vi "FFT no clk.vi"() -> ()   [LabVIEW 2014]
uses:
  <vilib>/Platform/TimedLoop/XDataNode/timing_clust.ctl
  <vilib>/Platform/TimedLoop/XDataNode/nitl_modes.ctl
  <vilib>/Platform/TimedLoop/XDataNode/wakeup.ctl
  <vilib>/rvi/Analysis/measure/FFT/simModelSupport/niFPGA FFT Streaming Sim Properties.ctl
  <vilib>/rvi/Analysis/measure/FFT/simModelSupport/niFPGA FFT Sim Stream Group Properties.ctl
  <vilib>/rvi/Analysis/measure/FFT/simModelSupport/niFPGA FFT Sim Types.ctl
  <vilib>/rvi/Analysis/measure/FFT/simModelSupport/niFpgaFFTSimArithmeticProperties.ctl
  <vilib>/rvi/Analysis/measure/FFT/simModelSupport/niFpgaFFTSimDfxp.ctl
  <vilib>/fxp/LVFixedPointQuantizationPolicyTypeDef.ctl
  <vilib>/rvi/Analysis/measure/FFT/XNode/niFpgaFFTButterflyDelays.ctl
  <vilib>/rvi/Emulation/niFpgaSctlEmulationGetInTimedLoop.vi
  <vilib>/rvi/Emulation/niFpgaEmulationReportErrorSimple.vi
  <vilib>/rvi/Emulation/niFpgaGetClockAttributes.vi
  <vilib>/rvi/Emulation/niFpgaCriticalErrorInLSC.vi
  <vilib>/rvi/Emulation/niFpgaEmulationIsFPGAContextNoSignature.vi
  <vilib>/rvi/errors/niFpgaSetErrorForExecOnDevCompSimple.vi
  <vilib>/rvi/eio/common/nirviEmuReportErrorAndStop.vi
  <vilib>/rvi/DataTransferAndStorage/Container/Common/niFpgaContainerGetUniqueNameForEmu.vi
  <vilib>/rvi/FIFO/Fifo_Resource/nirvififoEmulationSetSize.vi
  <vilib>/rvi/FIFO/Fifo_Resource/nirviFifoEmulationQueueMgr.vi
  <instcachedir>/0/nirviFifoEmulationQueueMgr_E5CAEC123FF24DC58D834DCA3CDAA9B5.lvgen/nirviFifoEmulationQueueMgr_E5CAEC123FF24DC58D834DCA3CDAA9B5_011.vi
  <vilib>/rvi/FIFO/Fifo_Resource/nirvififoEmulationCreateLock.vi
  <vilib>/rvi/Emulation/niFpgaProcessEmulError.vi
  <vilib>/rvi/FIFO/Fifo_Resource/nirvififoEmulationObtainLock.vi
  <vilib>/rvi/FIFO/Fifo_Resource/nirvififoEmulationReleaseLock.vi
  <vilib>/rvi/occurrence/nirviWaitOnOccurrenceBase.vi
  <vilib>/rvi/errors/nirviReportUnexpectedCaseInternalError.vi
  <vilib>/rvi/errors/nirviReportUnexpectedCaseInternalError (U32).vi
  <vilib>/rvi/Memory/Memory_Emulation/niFpgaMemoryEmulationCacheClearOnFirstRun.vi
  <vilib>/rvi/Memory/Memory_Emulation/nirvimemoryEmulationManagerCache_MakeExclusive.vi
  <vilib>/rvi/Memory/Memory_Emulation/niFpgaMemoryEmulationValidateCache.vi
  <vilib>/rvi/Memory/Memory_Emulation/nirvimemoryEmulationManagerCache_InsertValue.vi
  <vilib>/Utility/error.llb/Clear Errors.vi
  <vilib>/rvi/Memory/Memory_Emulation/nirvimemoryEmulationManagerCache_ReleaseExclusive.vi
  <vilib>/rvi/Memory/Memory_Emulation/nirvimemoryEmulationManagerCache_GetValue.vi
  <vilib>/rvi/Memory/Memory_Emulation/nirvimemoryEmulationManagerCache_SetValue.vi
  <instcachedir>/0/nirviFifoEmulationQueueMgr_E5CAEC123FF24DC58D834DCA3CDAA9B5.lvgen/nirviFifoEmulationQueueMgr_E5CAEC123FF24DC58D834DCA3CDAA9B5_010.vi
  <vilib>/rvi/FIFO/Fifo_Resource/nirvififoEmulationDetermineInputValidOut.vi
  <vilib>/rvi/Memory/Memory_Emulation/nirvimemoryFastEmulation.vi
  <vilib>/rvi/Memory/Memory_Emulation/nirvimemoryEmulation.vi
  <vilib>/rvi/Analysis/measure/FFT/simModelSupport/niFpgaFFTSimModelStreamingCore.vi
  <vilib>/rvi/eio/common/nirviEmuTemplateMethod_errors.vi
  <vilib>/Platform/TimedLoop/XDataNode/XDataNode.xnode
  <vilib>/rvi/DataTransferAndStorage/Container/XNode/niFpgaContainer.xnode
  <vilib>/rvi/FIFO/Fifo_Resource/nirvififoEmulationRead.vi
  <vilib>/rvi/DataTransferAndStorage/Register/Emulation/niFpgaRegisterEmulation.vi
  <vilib>/rvi/FIFO/Fifo_Resource/nirvififoEmulationWrite.vi
  <vilib>/rvi/FIFO/Fifo_Resource/nirvififoEmulationGetNumberOfElementsToWrite.vi
  <vilib>/rvi/Analysis/measure/FFT/XNode/niFpgaFFT.xnode
  <vilib>/eio/EIOMethodNode/EIOMethodNode.xnode
  <vilib>/Platform/TimedLoop/XDataNode/XDNodeRunTimeDep.lvlib
panel:
  in  "first bin":i32=4
  in  "last bin":i32=251
  in  "lower limit 2":u32=682
  in  "lower limit 1":u32=57
  in  "upper limit 2":u32=1194
  in  "upper limit 1":u32=569
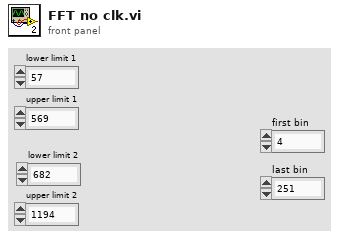
[diagram p1: front panel]
types:
  T1 = typedef "XDNodeRunTimeDep.lvlib/timing_clust.ctl" = cluster{"Expected End [f-1]":u64, "Actual End [f-1]":u64, "Finished Late? [f-1]":bool, "Expected End [i-1]":u64, "Actual End [i-1]":u64, "Finished Late? [i-1]":bool, "Expected Start [i]":u64, "Actual Start [i]":u64, "Expected Start [f]":u64, "Actual Start [f]":u64, "Source Name":string, "Structure Name":string, "Period":i64, "Deadline":i64, "Offset":i64, "Start":i64, "Priority":i32, "Timeout":i32, "Mode":T2, "Wakeup Reason":T3, "Error":errorcluster, "Source Type":string, "Secondary Source Type":string, "Global End Time":u64, "Global Start Time":u64, "Frame Duration":u64, "Iteration Duration":u64, "Assigned CPU":i32, "I/O Scan Engine Mode":u32}
  T2 = typedef "XDNodeRunTimeDep.lvlib/nitl_modes.ctl" = enum32{"No Change", "Process missed periods, maintain original phase", "Discard missed periods, maintain original phase", "Process missed periods, ignore original phase", "Discard missed periods, ignore original phase"}
  T3 = typedef "XDNodeRunTimeDep.lvlib/wakeup.ctl" = enum32{"Normal", "Aborted", "Asynchronous wakeup", "Timing source error", "Timed loop error", "Timeout"}
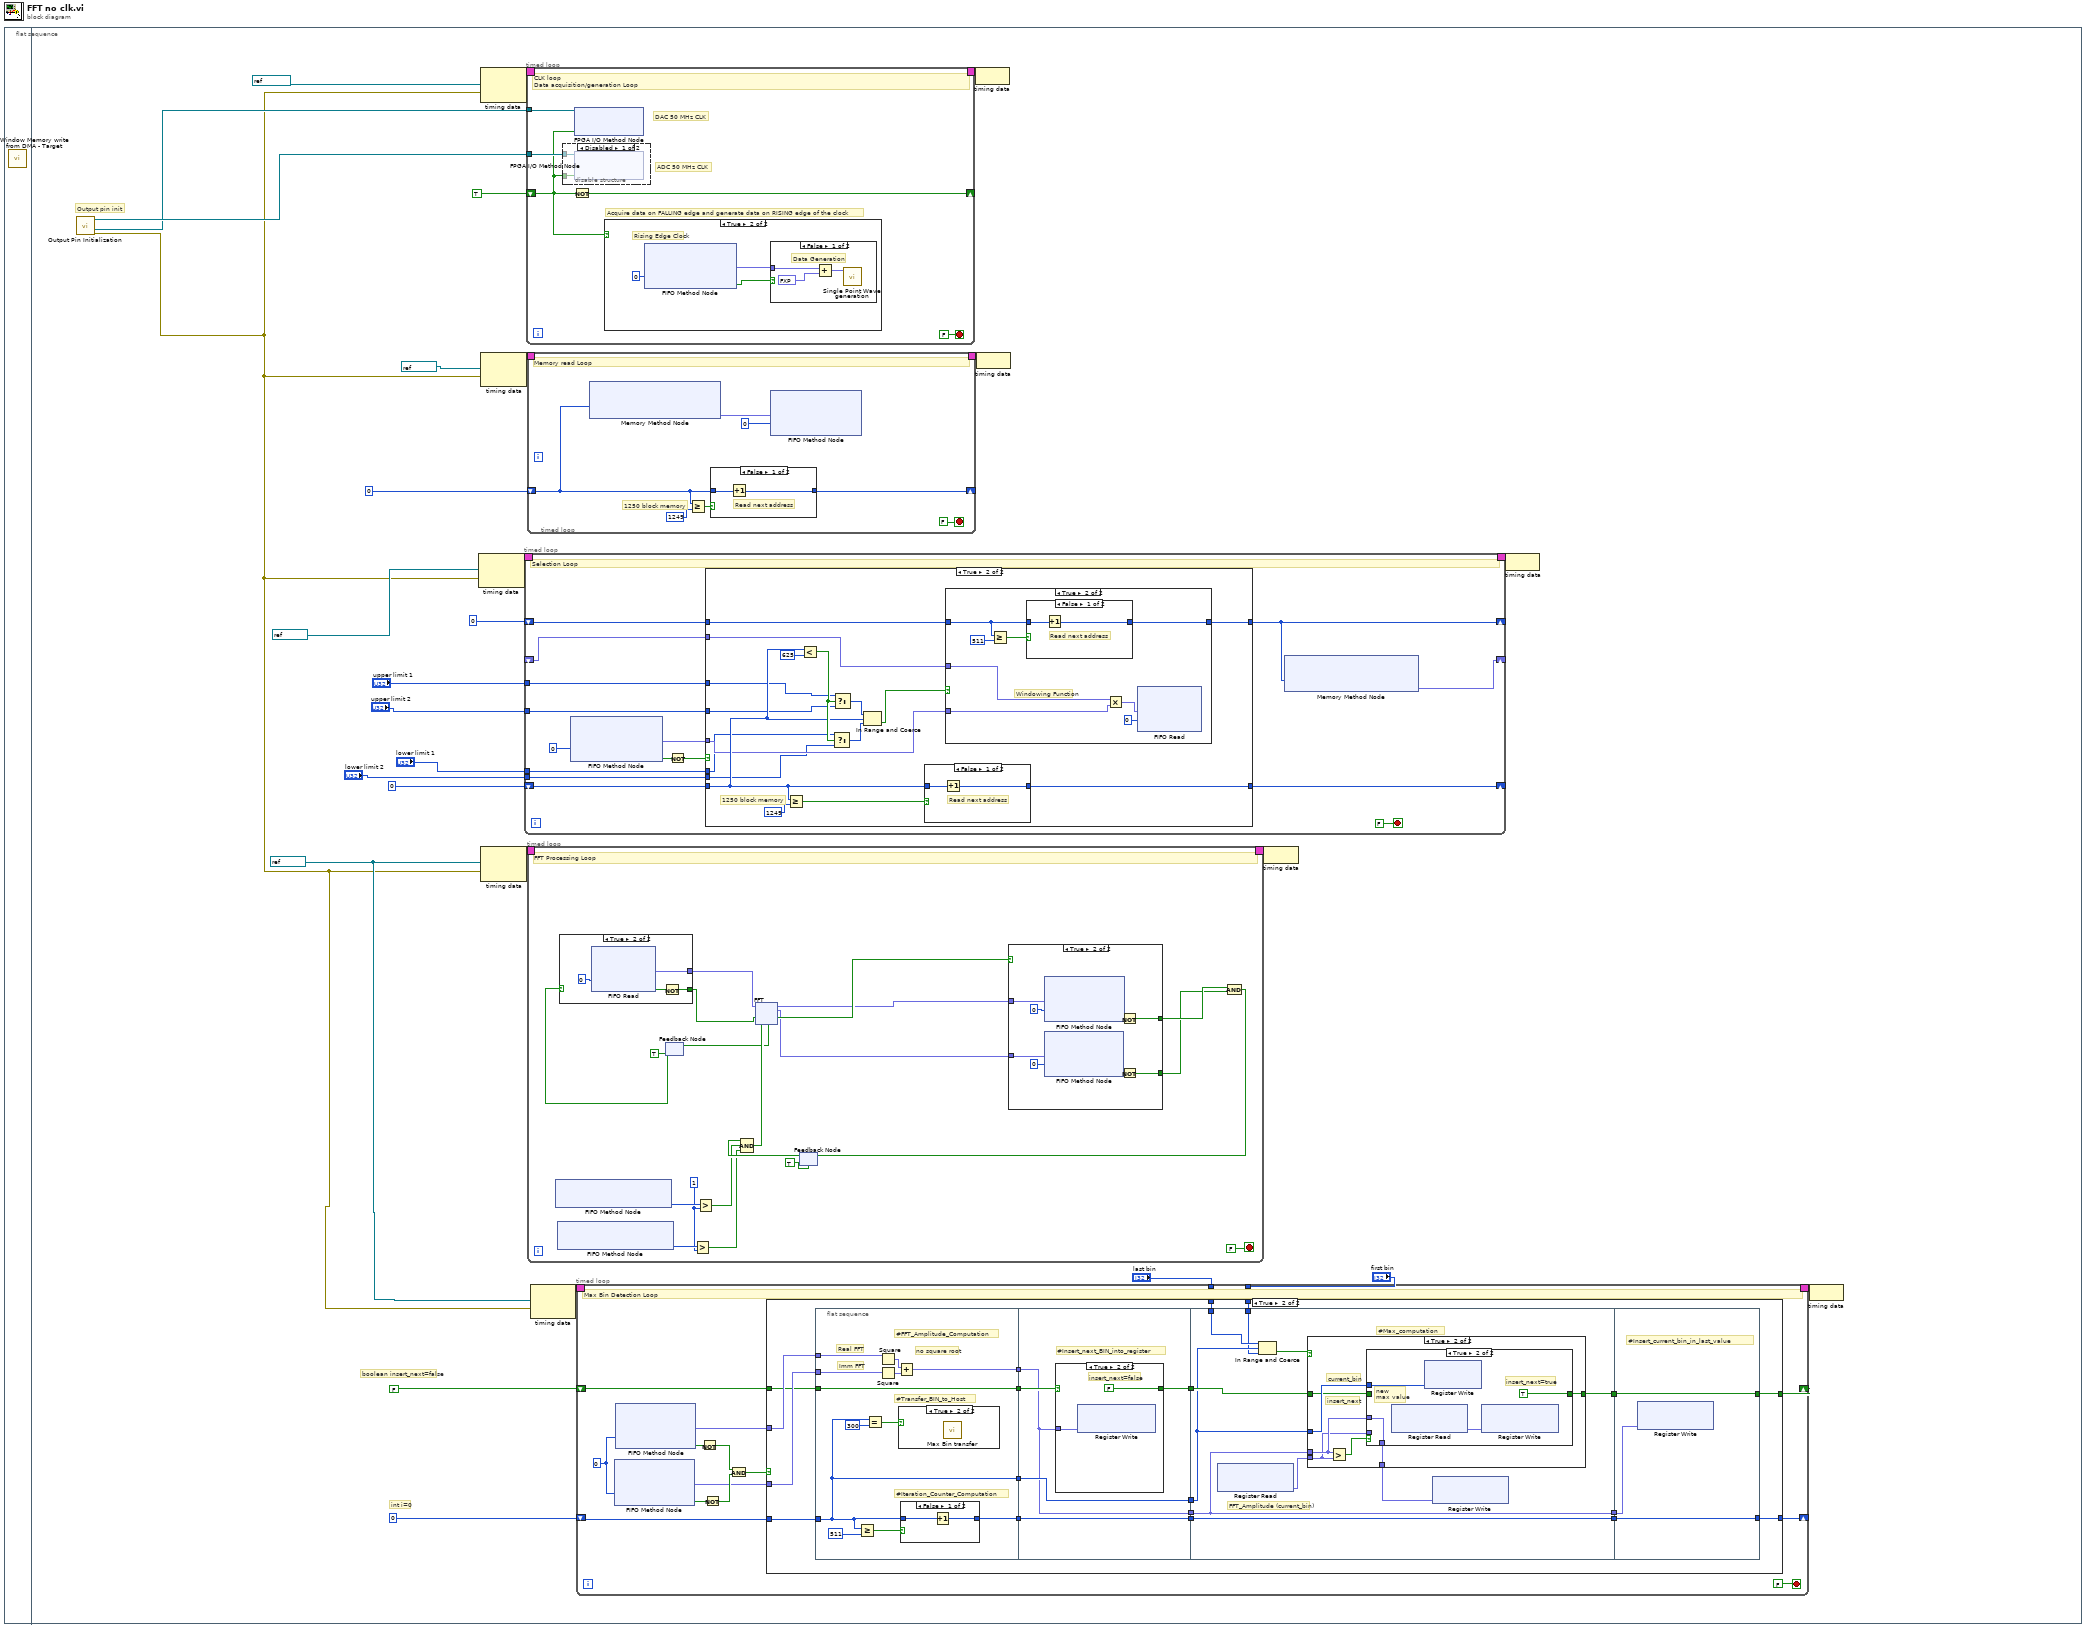
[diagram p0: block diagram]
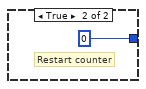
[diagram p4: hidden frame]
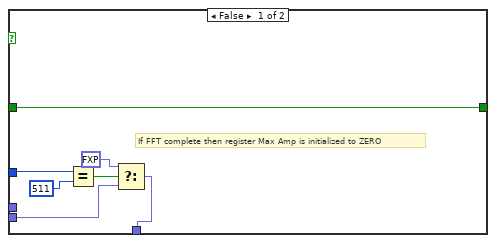
[diagram p6: hidden frame]
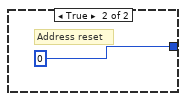
[diagram p10: hidden frame]
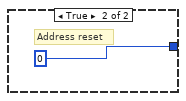
[diagram p11: hidden frame]
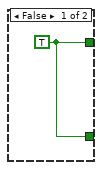
[diagram p12: hidden frame]
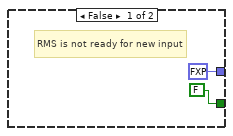
[diagram p13: hidden frame]
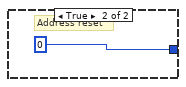
[diagram p14: hidden frame]
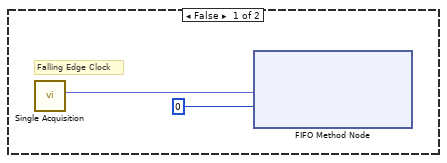
[diagram p16: hidden frame]
diagram:
  n1 = flat-sequence {
    frame #0 {
      n2 = call "Window Memory write from DMA - Target.vi"() -> ()  [unwired: 12 in]
    }
    frame #1 {
      w9 = refnum<k21> "50MHz" ("Source Name")
      # "int i=0"
      # "boolean insert_next=false"
      # "Output pin init"
      n3 = call "Output Pin Initialization.vi"() -> ("error out"=w8:errorcluster, "I/O Out Clock DAC (pin16)"=w14:refnum<k21>, "I/O Out Clock ADC (pin17)"=w15:refnum<k21>)  [unwired: 8 in]
      n4 = node-c288(refnum<k21> "50MHz" ("Source Name"), w8) -> (w23:T1)
      n5 = node-c288(refnum<k21> "100MHz" ("Source Name"), w8) -> (w29:T1)
      n6 = node-c288(refnum<k21> "50MHz" ("Source Name"), w8) -> (w27:T1)
      n7 = node-c288(w9, w8) -> (w25:T1)
      n8 = timed-loop {
        timing: w23 -> [_]
        timing-out: [_] -> w22
        shift-right: [w142] -> _
        shift-left: u32 0 -> [w141]
        tunnel: "upper limit 1" -> [w136]
        tunnel: "upper limit 2" -> [w135]
        tunnel: "lower limit 1" -> [w134]
        tunnel: "lower limit 2" -> [w133]
        shift-right: [w129] -> _
        shift-left: u32 0 -> [w132]
        shift-right: [w130] -> _
        shift-left: _ -> [w131]
        stop <- FALSE stop-if-true
        # "Selection Loop"
        n9 = xnode ("FIFO Method Node")("Timeout"=0) -> ("Element"=w138:fxp<+/-,12,12>, "Timed Out?"=w139:bool)  [unwired: 1 in, 1 out]
        n10 = Not(x=w139) -> (.not. x?=w140:bool)
        n11 = case shown="True" w140 {
          tunnel: [w145 w160] -> w142
          tunnel: w141 -> [w145 w155]
          tunnel: w138 -> [_ w153]
          tunnel: w136 -> [_ w152]
          tunnel: w135 -> [_ w151]
          tunnel: w134 -> [_ w150]
          tunnel: w133 -> [_ w149]
          tunnel: w132 -> [w144 w146]
          tunnel: [w144 w148] -> w129
          tunnel: w131 -> [_ w147]
          frame False {
          }
          frame True {
            # "1250 block memory"
            n12 = Greater Or Equal?(x=w155, y=u32 1249) -> (x >= y?=w161:bool)
            n13 = Less?(x=w155, y=u32 625) -> (x < y?=w156:bool)
            n14 = Select(t=w150, s=w156, f=w149) -> (s? t:f=w158:u32)
            n15 = Select(t=w152, s=w156, f=w151) -> (s? t:f=w159:u32)
            n16 = In Range and Coerce(upper limit=w159, x=w155, lower limit=w158) -> (In Range?=w154:bool)  [unwired: 1 out]
            n17 = case shown="False" w161 {
              tunnel: w155 -> [w176 _]
              tunnel: [w175 u32 0] -> w160
              frame False {
                # "Read next address"
                n18 = Increment(x=w176) -> (x+1=w175:u32)
              }
              frame True {
                # "Address reset"
              }
            }
            n19 = case shown="True" w154 {
              tunnel: w153 -> [_ w170]
              tunnel: w146 -> [w163 w166]
              tunnel: [w163 w168] -> w148
              tunnel: w147 -> [_ w164]
              frame False {
              }
              frame True {
                # "Windowing Function"
                n20 = Greater Or Equal?(x=w166, y=u32 511) -> (x >= y?=w167:bool)
                n21 = case shown="False" w167 {
                  tunnel: w166 -> [w173 _]
                  tunnel: [w172 u32 0] -> w168
                  frame False {
                    # "Read next address"
                    n22 = Increment(x=w173) -> (x+1=w172:u32)
                  }
                  frame True {
                    # "Address reset"
                  }
                }
                n23 = Multiply(x=w164, y=w170) -> (x*y=w169:fxp<+/-,12,12>)
                n24 = xnode ("FIFO Read")("Element"=w169, "Timeout"=0) -> ()  [unwired: 1 in, 2 out]
              }
            }
          }
        }
        n25 = xnode ("Memory Method Node")("Address"=w129) -> ("Data"=w130:fxp<+,8,1>)  [unwired: 1 in, 1 out]
      }
      n26 = timed-loop {
        timing: w29 -> [_]
        timing-out: [_] -> w28
        shift-right: [w272] -> _
        shift-left: TRUE -> [w270]
        tunnel: w14 -> [w274]
        tunnel: w15 -> [w271]
        stop <- FALSE stop-if-true
        # "ADC 50 MHz CLK"
        # "DAC 50 MHz CLK"
        # "Acquire data on FALLING edge and generate data on RISING edge of the clock"
        # "CLK loop\nData acquisition/generation Loop"
        n27 = disable-structure shown="Disabled" {
          disable-tunnel: w271 -> [w276 _]
          disable-tunnel: w270 -> [w275 _]
          frame Disabled {
            n28 = xnode "FPGA I/O Method Node"("FPGA I/O In"=w276, "Data"=w275) -> ()  [unwired: 1 out]
          }
          frame Enabled {
          }
        }
        n29 = Not(x=w270) -> (.not. x?=w272:bool)
        n30 = xnode "FPGA I/O Method Node"("FPGA I/O In"=w274, "Data"=w270) -> ()  [unwired: 1 out]
        n31 = case shown="True" w270 {
          frame False {
            # "Falling Edge Clock"
            n32 = call "Single Acquisition.vi"() -> ("Out"=w278:fxp<+/-,12,12>)  [unwired: 10 in, 1 out]
            n33 = xnode ("FIFO Method Node")("Element"=w278, "Timeout"=0) -> ()  [unwired: 1 in, 2 out]
          }
          frame True {
            # "Rising Edge Clock"
            n34 = xnode ("FIFO Method Node")("Timeout"=0) -> ("Element"=w279:fxp<+/-,12,12>, "Timed Out?"=w280:bool)  [unwired: 1 in, 1 out]
            n35 = case shown="False" w280 {
              tunnel: w279 -> [w284 _]
              frame False {
                # "Data Generation"
                n36 = Add(x=w284, y=fxp<+,12,12> 2048.0) -> (x+y=w282:fxp<+/-,14,14>)
                n37 = call "Single Point Wave generation.vi"("Data To Write"=w282) -> ()  [unwired: 10 in, 1 out]
              }
              frame True {
                # "FPGA memory slow"
              }
            }
          }
        }
      }
      n38 = timed-loop {
        timing: w27 -> [_]
        timing-out: [_] -> w26
        shift-right: [w257] -> _
        shift-left: u32 0 -> [w255]
        stop <- FALSE stop-if-true
        # "1250 block memory"
        # "Memory read Loop"
        n39 = xnode ("Memory Method Node")("Address"=w255) -> ("Data"=w254:fxp<+/-,12,12>)  [unwired: 1 in, 1 out]
        n40 = Greater Or Equal?(x=w255, y=u32 1249) -> (x >= y?=w258:bool)
        n41 = case shown="False" w258 {
          tunnel: w255 -> [w261 _]
          tunnel: [w260 u32 0] -> w257
          frame False {
            # "Read next address"
            n42 = Increment(x=w261) -> (x+1=w260:u32)
          }
          frame True {
            # "Address reset"
          }
        }
        n43 = xnode ("FIFO Method Node")("Element"=w254, "Timeout"=0) -> ()  [unwired: 1 in, 2 out]
      }
      n44 = timed-loop {
        timing: w25 -> [_]
        timing-out: [_] -> w24
        stop <- FALSE stop-if-true
        w187 = u32 1 ("y")
        # "FFT Processing Loop"
        n45 = xnode ("FIFO Method Node")() -> ("Number of Elements to Write"=w189:u32)  [unwired: 1 in, 1 out]
        n46 = xnode ("FIFO Method Node")() -> ("Number of Elements to Write"=w188:u32)  [unwired: 1 in, 1 out]
        n47 = feedback #1(TRUE ("ready for input")) -> (w204:bool)
        n48 = case shown="True" w204 {
          tunnel: [FALSE w245] -> w198
          tunnel: [fxp<+/-,12,12> 0.0 ("Element") w242] -> w199
          frame False {
            # "RMS is not ready for new input"
          }
          frame True {
            n49 = xnode ("FIFO Read")("Timeout"=0) -> ("Element"=w242:fxp<+/-,12,12>, "Timed Out?"=w244:bool)  [unwired: 1 in, 1 out]
            n50 = Not(x=w244) -> (.not. x?=w245:bool)
          }
        }
        n51 = Greater?(x=w188, y=w187) -> (0:w185:bool)
        n52 = Greater?(x=w189, y=w187) -> (0:w186:bool)
        n53 = feedback #2(TRUE) -> (w200:bool)
        n54 = Compound Arithmetic op=AND(w200, w186, w185) -> (w197:bool)
        n55 = xnode "FFT"("real data in"=w199, "input valid"=w198, "ready for output"=w197) -> ("ready for input"=w196:bool, "real data out"=w194:fxp<+/-,22,22>, "imaginary data out"=w193:fxp<+/-,22,22>, "output valid"=w195:bool)  [unwired: 2 in, 1 out]
        n56 = feedback-in #1(w196) -> ()
        n57 = case shown="True" w195 {
          tunnel: w194 -> [_ w239]
          tunnel: w193 -> [_ w238]
          tunnel: [w231 w237] -> w192
          tunnel: [w231 w236] -> w191
          frame False {
            w231 = TRUE
          }
          frame True {
            n58 = xnode ("FIFO Method Node")("Element"=w239, "Timeout"=0) -> ("Timed Out?"=w232:bool)  [unwired: 1 in, 1 out]
            n59 = xnode ("FIFO Method Node")("Element"=w238, "Timeout"=0) -> ("Timed Out?"=w233:bool)  [unwired: 1 in, 1 out]
            n60 = Not(x=w232) -> (.not. x?=w237:bool)
            n61 = Not(x=w233) -> (.not. x?=w236:bool)
          }
        }
        n62 = Compound Arithmetic op=AND(w192, w191) -> (w190:bool)
        n63 = feedback-in #2(w190) -> ()
      }
      n64 = node-c288(w9, w8) -> (w21:T1)
      n65 = timed-loop {
        shift-right: [w35] -> _
        shift-left: 0 ("Timeout") -> [w36]
        shift-right: [w33] -> _
        shift-left: FALSE -> [w34]
        timing: w21 -> [_]
        timing-out: [_] -> w20
        tunnel: "last bin" -> [w31]
        tunnel: "first bin" -> [w30]
        stop <- FALSE stop-if-true
        w44 = 0 ("Timeout")
        # "Max Bin Detection Loop"
        n66 = xnode ("FIFO Method Node")("Timeout"=w44) -> ("Element"=w37:fxp<+/-,22,22>, "Timed Out?"=w42:bool)  [unwired: 1 in, 1 out]
        n67 = xnode ("FIFO Method Node")("Timeout"=w44) -> ("Element"=w38:fxp<+/-,22,22>, "Timed Out?"=w43:bool)  [unwired: 1 in, 1 out]
        n68 = Not(x=w43) -> (.not. x?=w41:bool)
        n69 = Not(x=w42) -> (.not. x?=w40:bool)
        n70 = And(x=w41, y=w40) -> (x .and. y?=w39:bool)
        n71 = case shown="True" w39 {
          tunnel: w38 -> [_ w65]
          tunnel: w37 -> [_ w64]
          tunnel: w36 -> [w46 w62]
          tunnel: [w46 w49] -> w35
          tunnel: w34 -> [w45 w56]
          tunnel: [w45 w51] -> w33
          tunnel: w31 -> [_ w48]
          tunnel: w30 -> [_ w47]
          frame False {
            # "Data are NOT ready in Target Real FFT and Target Imm FFT FIFOs"
          }
          frame True {
            n72 = flat-sequence {
              tunnel: w65 -> [w74]
              tunnel: w64 -> [w75]
              tunnel: [w73] -> w63
              tunnel: w62 -> [w66]
              tunnel: [w72] -> w61
              tunnel: [w66] -> w58
              tunnel: [w69] -> w57
              tunnel: w56 -> [w69]
              tunnel: w63 -> [w82]
              tunnel: w61 -> [w85]
              tunnel: [w85] -> w60
              tunnel: w58 -> [w83]
              tunnel: w57 -> [w84]
              tunnel: [w83] -> w55
              tunnel: [w82] -> w54
              tunnel: [w81] -> w53
              tunnel: w60 -> [w98]
              tunnel: [w98] -> w59
              tunnel: w55 -> [w93]
              tunnel: w54 -> [w95]
              tunnel: w53 -> [w96]
              tunnel: [w95] -> w52
              tunnel: [w94] -> w50
              tunnel: w48 -> [w90]
              tunnel: w47 -> [w89]
              tunnel: w59 -> [w119]
              tunnel: w52 -> [w121]
              tunnel: w50 -> [w120]
              tunnel: [w120] -> w51
              tunnel: [w119] -> w49
              frame #0 {
                # "no square root"
                # "#Transfer_BIN_to_Host"
                # "#Iteration_Counter_Computation"
                # "#FFT_Amplitude_Computation"
                # "Imm FFT"
                # "Real FFT"
                n73 = Greater Or Equal?(x=w66, y=511) -> (x >= y?=w70:bool)
                n74 = Equal?(x=w66, y=300) -> (x = y?=w68:bool)
                n75 = Square(x=w74) -> (x^2=w77:fxp<+,43,43>)
                n76 = Square(x=w75) -> (x^2=w76:fxp<+,43,43>)
                n77 = Add(x=w77, y=w76) -> (x+y=w73:fxp<+,44,44>)
                n78 = case shown="True" w68 {
                  frame False {
                    # "FFT Comp is NOT finished"
                  }
                  frame True {
                    n79 = call "Max Bin transfer.vi"() -> ()  [unwired: 11 in, 1 out]
                  }
                }
                n80 = case shown="False" w70 {
                  tunnel: w66 -> [w78 _]
                  tunnel: [w79 0 ("Timeout")] -> w72
                  frame False {
                    n81 = Increment(x=w78) -> (x+1=w79:i32)
                  }
                  frame True {
                    # "Restart counter"
                  }
                }
              }
              frame #1 {
                # "#Insert_next_BIN_into_register"
                n82 = case shown="True" w84 {
                  selector: w84 -> [w86 _]
                  tunnel: [w86 FALSE] -> w81
                  tunnel: w82 -> [_ w87]
                  frame False {
                  }
                  frame True {
                    # "insert_next=false"
                    n83 = xnode ("Register Write")("Data"=w87) -> ()  [unwired: 1 in, 1 out]
                  }
                }
              }
              frame #2 {
                # "FFT_Amplitude (current_bin)"
                # "#Max_computation"
                n84 = xnode ("Register Read")() -> ("Data"=w92:fxp<+,44,44>)  [unwired: 1 in, 1 out]
                n85 = In Range and Coerce(upper limit=w90, x=w93, lower limit=w89) -> (In Range?=w97:bool)  [unwired: 1 out]
                n86 = case shown="True" w97 {
                  tunnel: w95 -> [_ w111]
                  tunnel: w93 -> [w103 w110]
                  tunnel: w96 -> [w105 w109]
                  tunnel: [w105 w108] -> w94
                  tunnel: w92 -> [w101 w106]
                  tunnel: [w99 w107] -> w91
                  frame False {
                    # "If FFT complete then register Max Amp is initialized to ZERO"
                    n87 = Equal?(x=w103, y=511) -> (x = y?=w104:bool)
                    n88 = Select(t=fxp<+,44,44> 0.0, s=w104, f=w101) -> (s? t:f=w99:fxp<+,44,44>)
                  }
                  frame True {
                    # "insert_next"
                    # "current_bin"
                    n89 = Greater?(x=w111, y=w106) -> (0:w112:bool)
                    n90 = case shown="True" w112 {
                      tunnel: w111 -> [_ w115]
                      tunnel: w110 -> [_ w118]
                      tunnel: w109 -> [w114 _]
                      tunnel: [w114 TRUE] -> w108
                      tunnel: [w113 w115] -> w107
                      tunnel: w106 -> [w113 _]
                      frame False {
                        # "Old value is re-written"
                      }
                      frame True {
                        # "new\nmax value"
                        # "insert_next=true"
                        n91 = xnode ("Register Read")() -> ("Data"=w116:fxp<+,44,44>)  [unwired: 1 in, 1 out]
                        n92 = xnode ("Register Write")("Data"=w118) -> ()  [unwired: 1 in, 1 out]
                        n93 = xnode ("Register Write")("Data"=w116) -> ()  [unwired: 1 in, 1 out]
                      }
                    }
                  }
                }
                n94 = xnode ("Register Write")("Data"=w91) -> ()  [unwired: 1 in, 1 out]
              }
              frame #3 {
                # "#Insert_current_bin_in_last_value"
                n95 = xnode ("Register Write")("Data"=w121) -> ()  [unwired: 1 in, 1 out]
              }
            }
          }
        }
      }
      n96 = node-c288(w28) -> ()
      n97 = node-c288(w26) -> ()
      n98 = node-c288(w24) -> ()
      n99 = node-c288(w22) -> ()
      n100 = node-c288(w20) -> ()
    }
  }
